vi "_Update Ramping Experiment.vi"(4 "Ramping Ch":T1[](array[typedef]), 5 "error in":errorcluster, 6 "Offset":u16, 7 "Expt":T2 {"Mass Range"."Resolution Type" items=["High/High", "Medium/Medium", "Low/Low", "High/Medium", "High/Low", "Medium/High", "Medium/Low", "Low/High", "Low/Medium"]}) -> (0 "error out":errorcluster, 1 "Next Offset":u16)   [LabVIEW 2015]
uses:
  Type/_RT Expt.ctl
  Type/_Run Mode.ctl
  Type/_RT Active Ch.ctl
  Type/_RT Mass Range.ctl
  Type/_RT Res Type.ctl
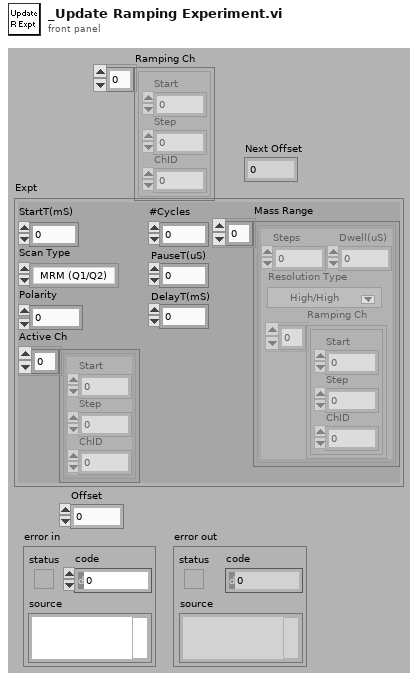
[diagram p1: front panel]
types:
  T1 = typedef "_RT Active Ch.ctl" = cluster{"Start":i32, "Step":i32, "ChID":i32}
  T2 = typedef "_RT Expt.ctl" = cluster{"StartT(mS)":i32, "#Cycles":i32, "Scan Type":T3, "PauseT(uS)":i32, "Polarity":u8, "DelayT(mS)":i32, "Active Ch":T1[], "Mass Range":T4[]}
  T3 = typedef "_Run Mode.ctl" = enum16{"MRM (Q1/Q2)", "Q1 Scan", "Q1 SRM", "Q2 Scan", "Q2 SRM", "Product Scan", "Precursor Scan", "Neutral Loss", "Neutral Gain"}
  T4 = typedef "_RT Mass Range.ctl" = cluster{"Steps":i32, "Dwell(uS)":i32, "Resolution Type":T5, "Ramping Ch":T1[]}
  T5 = typedef "_RT Res Type.ctl" = u16
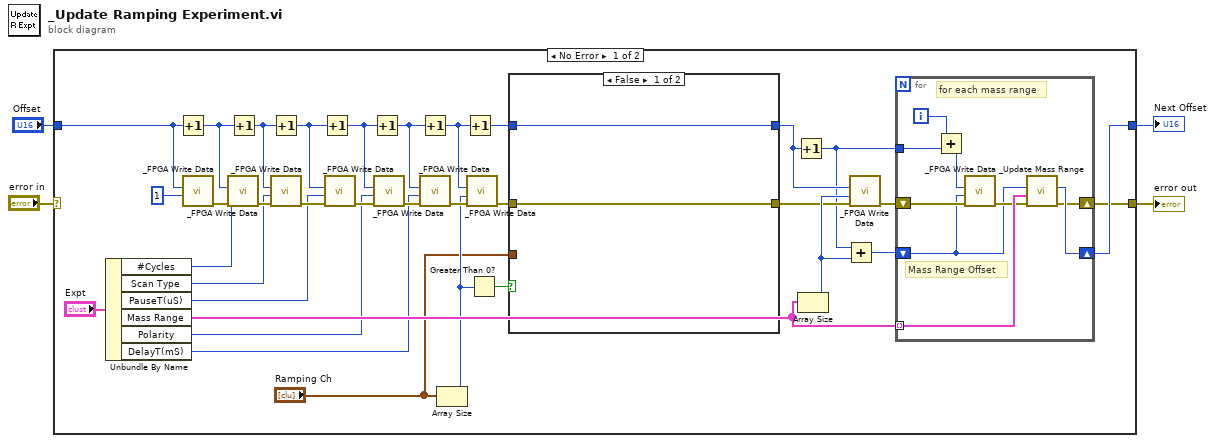
[diagram p0: block diagram]
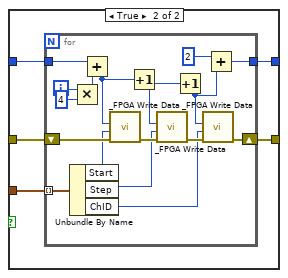
[diagram p2: hidden frame]
diagram:
  n1 = case shown="No Error" "error in" {
    selector: "error in" -> [_ w73]
    tunnel: [w29 w73] -> w3
    tunnel: "Offset" -> [w31 w72]
    tunnel: [w30 w72] -> w1
    frame No Error {
      n2 = Unbundle By Name("Expt") -> ("#Cycles"=w36:i32, "Scan Type"=w21:T3, "PauseT(uS)"=w17:i32, "Mass Range"=w32:T4[], "Polarity"=w16:u8, "DelayT(mS)"=w13:i32)
      n3 = Increment(x=w31) -> (x+1=w35:u16)
      n4 = call "_FPGA Write Data.vi"("Data"=u32 1, "Address"=w31) -> ("error out"=w37:errorcluster)  [unwired: 4 in, 2 out]
      n5 = call "_FPGA Write Data.vi"("error in"=w37, "Data"=w36, "Address"=w35) -> ("error out"=w26:errorcluster)  [unwired: 3 in, 2 out]
      n6 = Increment(x=w35) -> (x+1=w25:u16)
      n7 = Increment(x=w25) -> (x+1=w18:u16)
      n8 = call "_FPGA Write Data.vi"("error in"=w26, "Data"=w21, "Address"=w25) -> ("error out"=w20:errorcluster)  [unwired: 3 in, 2 out]
      n9 = Increment(x=w18) -> (x+1=w15:u16)
      n10 = call "_FPGA Write Data.vi"("error in"=w20, "Data"=w17, "Address"=w18) -> ("error out"=w19:errorcluster)  [unwired: 3 in, 2 out]
      n11 = Increment(x=w15) -> (x+1=w23:u16)
      n12 = call "_FPGA Write Data.vi"("error in"=w19, "Data"=w16, "Address"=w15) -> ("error out"=w22:errorcluster)  [unwired: 3 in, 2 out]
      n13 = Increment(x=w23) -> (x+1=w27:u16)
      n14 = call "_FPGA Write Data.vi"("error in"=w22, "Data"=w13, "Address"=w23) -> ("error out"=w28:errorcluster)  [unwired: 3 in, 2 out]
      n15 = Array Size(array="Ramping Ch") -> (size(s)=w9:i32)
      n16 = Increment(x=w27) -> (x+1=w11:u16)
      n17 = call "_FPGA Write Data.vi"("error in"=w28, "Data"=w9, "Address"=w27) -> ("error out"=w12:errorcluster)  [unwired: 3 in, 2 out]
      n18 = Greater Than 0?(x=w9) -> (x > 0?=w10:bool)
      n19 = case shown="False" w10 {
        tunnel: [w40 w42] -> w6
        tunnel: w12 -> [w40 w44]
        tunnel: w11 -> [w39 w43]
        tunnel: [w39 w41] -> w7
        tunnel: "Ramping Ch" -> [_ w45]
        frame False {
        }
        frame True {
          n20 = for {
            tunnel: w45 -> [w58] mode=indexing
            shift-right: [w50] -> w42
            shift-left: w44 -> [w57]
            tunnel: w43 -> [w59]
            tunnel: [w48] -> w41
            i -> [w62]
            n21 = Unbundle By Name(w58) -> ("Start"=w56:i32, "Step"=w46:i32, "ChID"=w51:i32)
            n22 = Multiply(x=w62, y=4) -> (x*y=w60:i32)
            n23 = Add(x=w59, y=w60) -> (x+y=w54:i32)
            n24 = call "_FPGA Write Data.vi"("error in"=w57, "Data"=w56, "Address"=w54) -> ("error out"=w55:errorcluster)  [unwired: 3 in, 2 out]
            n25 = Increment(x=w54) -> (x+1=w52:i32)
            n26 = call "_FPGA Write Data.vi"("error in"=w55, "Data"=w46, "Address"=w52) -> ("error out"=w53:errorcluster)  [unwired: 3 in, 2 out]
            n27 = Increment(x=w52) -> (x+1=w49:i32)
            n28 = call "_FPGA Write Data.vi"("error in"=w53, "Data"=w51, "Address"=w49) -> ("error out"=w50:errorcluster)  [unwired: 3 in, 2 out]
            n29 = Add(x=2, y=w49) -> (x+y=w48:i32)
          }
        }
      }
      n30 = Increment(x=w7) -> (x+1=w5:i32)
      n31 = Array Size(array=w32) -> (size(s)=w14:i32)
      n32 = Add(x=w5, y=w14) -> (x+y=w33:i32)
      n33 = call "_FPGA Write Data.vi"("error in"=w6, "Data"=w14, "Address"=w7) -> ("error out"=w34:errorcluster)  [unwired: 3 in, 2 out]
      n34 = for {
        shift-right: [w64] -> w29
        shift-left: w34 -> [w71]
        tunnel: w5 -> [w69]
        shift-right: [w65] -> w30
        shift-left: w33 -> [w66]
        tunnel: w32 -> [w68] mode=indexing
        i -> [w63]
        # "for each mass range"
        # "Mass Range Offset"
        n35 = Add(x=w63, y=w69) -> (x+y=w70:i32)
        n36 = call "_FPGA Write Data.vi"("error in"=w71, "Data"=w66, "Address"=w70) -> ("error out"=w67:errorcluster)  [unwired: 3 in, 2 out]
        n37 = call "_Update Mass Range.vi"("error in"=w67, "Mass Range"=w68, "Offset"=w66) -> ("error out"=w64:errorcluster, "Next Offset"=w65:u16)  [unwired: 1 in, 2 out]
      }
    }
    frame Error {
    }
  }
  "error out" <- w3
  "Next Offset" <- w1
